vi "keithley_output_control.vi"(8 "Source Mode  (0: Voltage)":u16(ring) items=["Voltage", "Current"], 9 "VISA resource name":refnum<visa-resource-name>, 10 "Compliance  Level (0.1)":dbl=0.1, 11 "Output Level (0)":dbl=1.0 format="%#_13g") -> (0 "VISA resource name out":refnum<visa-resource-name>, 1 "Current":sgl, 2 "Voltage":sgl)   [LabVIEW 2017]
uses:
  <instrlib>/keithley 24xx/Public/Data/Read (Single Point).vi
  <instrlib>/keithley 24xx/Keithley 24XX.lvlib
panel:
  in  "Serial Configuration":T1={"Baud Rate"=9600, "Parity"=0, "Data Bits"=8, "Stop Bits"=10, "Flow Control"=0} {"Flow Control" items=["None", "XON/XOFF", "RTS/CTS", "XON/XOFF & RTS/CTS", "DTR/DSR", "XON/XOFF & DTR/DSR"]; "Stop Bits" items=["1.0"=10, "1.5"=15, "2.0"=20]; "Data Bits" items=["7"=7, "8"=8]; "Parity" items=["None", "Odd", "Even", "Mark", "Space"]; "Baud Rate" items=["300"=300, "600"=600, "1200"=1200, "2400"=2400, "4800"=4800, "9600"=9600, "19200"=19200]}
  in  "Timeout (10000 ms)":i32=10000 format="%#.6g"
  # "(c) 2006 - 2015 National Instruments.  ALL RIGHTS RESERVED."
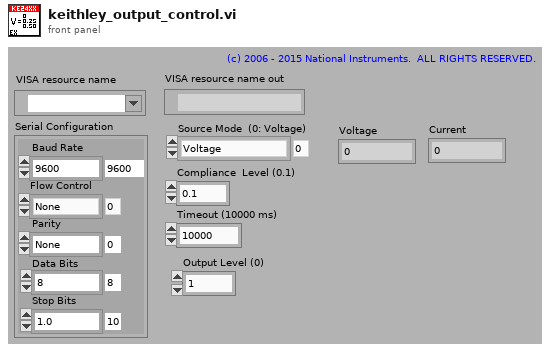
[diagram p1: front panel]
types:
  T1 = cluster{"Baud Rate":u32, "Parity":u16, "Data Bits":u16, "Stop Bits":u16, "Flow Control":u16}
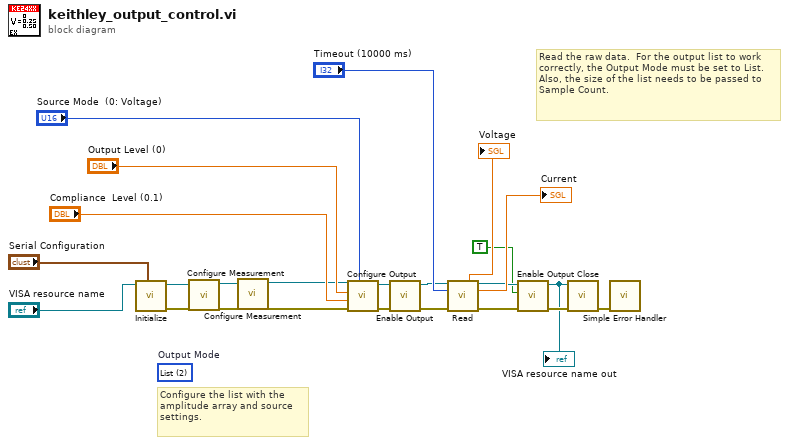
[diagram p0: block diagram]
diagram:
  (unwired) u16 2 items=["Fixed", "Sweep", "List"]  # Output Mode
  # "Read the raw data.  For the output list to work correctly, the Output Mode must be set to List.  Also, the size of the list needs to be passed to Sample Count."
  # "Configure the list with the amplitude array and source settings."
  n1 = call <instrlib>:"Initialize.vi"("Serial Configuration"="Serial Configuration", "VISA resource name"="VISA resource name") -> ("error out"=w4:errorcluster, "VISA resource name out"=w3:refnum<visa-resource-name>)  [unwired: 8 in]
  n2 = call <instrlib>:"Configure Measurement.vi"("error in (no error)"=w4, "VISA resource name"=w3) -> ("VISA resource name out"=w2:refnum<visa-resource-name>)  [unwired: 8 in, 1 out]
  n3 = call <instrlib>:"Configure Measurement.vi"("VISA resource name"=w2) -> ("VISA resource name out"=w1:refnum<visa-resource-name>)  [unwired: 9 in, 1 out]
  n4 = call <instrlib>:"Configure Output.vi"("Source Mode  (0: Voltage)"="Source Mode  (0: Voltage)", "error in (no error)"=w4, "Compliance  Level (0.1)"="Compliance  Level (0.1)", "Output Level (0)"="Output Level (0)", "VISA resource name"=w1) -> ("error out"=w9:errorcluster, "VISA resource name out"=w7:refnum<visa-resource-name>)  [unwired: 5 in]
  n5 = call <instrlib>:"Enable Output.vi"("error in (no error)"=w9, "VISA resource name"=w7) -> ("error out"=w15:errorcluster, "VISA resource name out"=w16:refnum<visa-resource-name>)  [unwired: 8 in]
  n6 = call-poly <instrlib>:"Read.vi"("VISA resource name"=w16, "Timeout (10000 ms)"="Timeout (10000 ms)", "error in (no error)"=w15) -> ("Voltage"=→"Voltage":sgl, "VISA resource name out"=w12:refnum<visa-resource-name>, "Current"=→"Current":sgl, "error out"=w11:errorcluster)  [unwired: 6 in, 3 out]
  n7 = call <instrlib>:"Enable Output.vi"("error in (no error)"=w11, "Enable Output (T: Enable)"=TRUE, "VISA resource name"=w12) -> ("error out"=w14:errorcluster, "VISA resource name out"=w13:refnum<visa-resource-name>)  [unwired: 7 in]
  "VISA resource name out" <- w13
  n8 = call <instrlib>:"Close.vi"("error in (no error)"=w14, "VISA resource name"=w13) -> ("error out"=w17:errorcluster)  [unwired: 9 in]
  n9 = call <vilib>:"Simple Error Handler.vi"("error in (no error)"=w17) -> ()  [unwired: 4 in, 5 out]
